vi "GetCurrViPath.vi"(2 "error in":errorcluster caption="错误输入", 3 "PathIn":path) -> (0 "error out":errorcluster caption="错误输出", 1 "CurrentViPath":path)   [LabVIEW 2013]
uses:
  GlobValue.vi
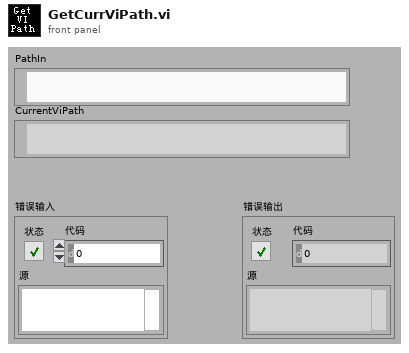
[diagram p1: front panel]
types:
  T1 = enum32{"invalid app kind", "Development System", "Run Time System", "Student Edition", "Embedded LabVIEW", "Evaluation", "Custom"}
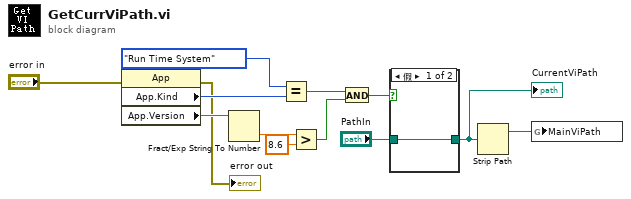
[diagram p0: block diagram]
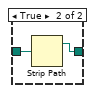
[diagram p2: hidden frame]
diagram:
  n1 = property class="App"(error in="error in") -> (error out=→"error out":errorcluster, "App.Kind"=w8:T1, "App.Version"=w9:string)  [unwired: 1 in, 1 out]
  n2 = Fract/Exp String To Number(string=w9) -> (number=w10:dbl)  [unwired: 4 out]
  n3 = Equal?(x=T1."Run Time System" ("y"), y=w8) -> (x = y?=w12:bool)
  n4 = Greater?(x=w10, y=8.6) -> (0:w13:bool)
  n5 = And(x=w12, y=w13) -> (x .and. y?=w6:bool)
  n6 = case shown="假" w6 {
    tunnel: [w14 w16] -> w4
    tunnel: "PathIn" -> [w14 w15]
    frame False {
    }
    frame True {
      n7 = Strip Path(path=w15) -> (stripped path=w16:path)  [unwired: 1 out]
    }
  }
  "CurrentViPath" <- w4
  n8 = Strip Path(path=w4) -> (stripped path=w3:path)  [unwired: 1 out]
  n9 = global write "GlobValue.vi" "MainViPath"(w3) -> ()
